vi "Method_Const.vi"(4 "Value":timestamp, 5 "Value A":refnum<class "Abs_Time.lvclass">) -> (1 "Result":refnum<class "Abs_Boolean.lvclass">)   [LabVIEW 2021, in "Less_Time.lvclass"]
uses:
  Less_Time.lvclass
  Abs_Types/Time/Abs_Time.lvclass
  Abs_Types/Boolean/Abs_Boolean.lvclass
  C:/TSA/LV_Abstract/Source/Functions/Support/Compare/Two Term/Time/AbsComp_Two Term_Time.lvclass
  C:/Program Files (x86)/National Instruments/LabVIEW 2021/vi.lib/TSA/Abstract Data Classes/Abs_Types/Boolean/Abs_Boolean.lvclass
  Support/Compare/Two Term/Time/AbsComp_Two Term_Time.lvclass/AbsComp_Two Term_Time.ctl
  Support/Compare/Two Term/Time/Properties/Write Time A.vi
  Support/Compare/Two Term/Time/Properties/Write Time B.vi
  Constants/Support/Time/Const_Time.lvclass
  C:/Program Files (x86)/National Instruments/LabVIEW 2021/vi.lib/TSA/Abstract Data Classes/Abs_Types/Time/Abs_Time.lvclass
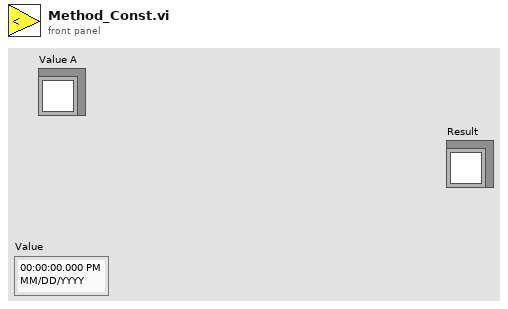
[diagram p1: front panel]
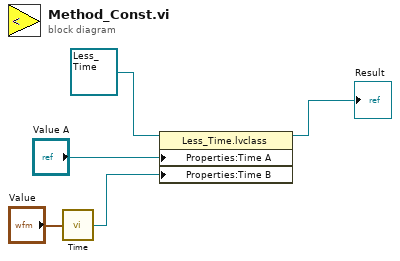
[diagram p0: block diagram]
diagram:
  n1 = call "Time.vi"("Value"="Value") -> ("Constant"=w2:refnum<class "Const_Time.lvclass">)  [unwired: 4 in]
  n2 = property class="Less_Time.lvclass"(reference=refnum<class "Less_Time.lvclass"> refnum ("Greater 0_U64.lvclass"), "Properties:Time A"="Value A", "Properties:Time B"=w2) -> (reference out=→"Result":refnum<class "Less_Time.lvclass">)  [unwired: 1 in, 1 out]
